vi "PC main.vi"() -> ()   [LabVIEW 2021]
uses:
  <vilib>/Platform/TimedLoop/XDataNode/wakeup.ctl
  <vilib>/Platform/TimedLoop/XDataNode/XDNodeRunTimeDep.lvlib
  <vilib>/Platform/TimedLoop/XDataNode/nitl_modes.ctl
  <vilib>/Platform/TimedLoop/XDataNode/timing_clust.ctl
  <vilib>/platform/TimedLoop/XDataNode/XDataNode.xnode
  <vilib>/RTI DDS Toolkit/Library/LVDDS_library.lvlib
  <vilib>/RTI DDS Toolkit/VIs/AdvancedCreateReader_NumI32.vi
  <vilib>/RTI DDS Toolkit/VIs/AdvancedCreateWriter_NumI32.vi
  <vilib>/RTI DDS Toolkit/Types/RTI DDS Advanced Writer Configuration.ctl
  <vilib>/RTI DDS Toolkit/Types/RTI DDS Advanced Reader Configuration.ctl
  <vilib>/RTI DDS Toolkit/VIs/Read_NumI32.vi
  <vilib>/RTI DDS Toolkit/VIs/Write_NumI32.vi
panel:
  in  "Record?":bool
  out "cluster":T1(graph)={"Numeric 4"=27.89473684210526, "Numeric 4"=27.105263157894736, "Numeric 4"=33.68421052631579}
  in  "Lock":bool
  in  "Python On":bool=TRUE
  in  "DDS On":bool
  out "Period":i64
  out "RBF Weights":dbl[](array[numeric])
  out "Robot Env":cluster{dbl[], dbl[]}[](graph)=[{[-0.02870597177988223], [-0.4509645928750905]}, {[-2.0, 2.0, 0.0], [-2.0, -2.0, 2.0]}, {[0.0], [0.0]}, {[0.0, 0.0, 0.0, 0.0, 0.0, 0.0, 0.0, 0.0, 0.0, -0.0, -0.0, -0.0, -0.0, -0.0, -0.0, -0.0, -0.0, -0.0, -0.0, -0.0, -0.0, -0.0, -0.0, -0.0, -0.0, 0.0, 0.0, 0.0, 0.0, 0.0, 0.0, 0.0], [0.0, 0.0, 0.0, 0.0, 0.0, 0.0, 0.0, 0.0, 0.0, 0.0, 0.0, 0.0, 0.0, 0.0, 0.0, 0.0, 0.0, -0.0, -0.0, -0.0, -0.0, -0.0, -0.0, -0.0, -0.0, -0.0, -0.0, -0.0, -0.0, -0.0, -0.0, -0.0]}]
  in  "Manual Control":dbl[](array[slide])=[27.89473684210526, 27.105263157894736, 33.68421052631579] scale=0.0..50.0
  in  "Manual Control":bool=TRUE
  in  "Host Stop":bool
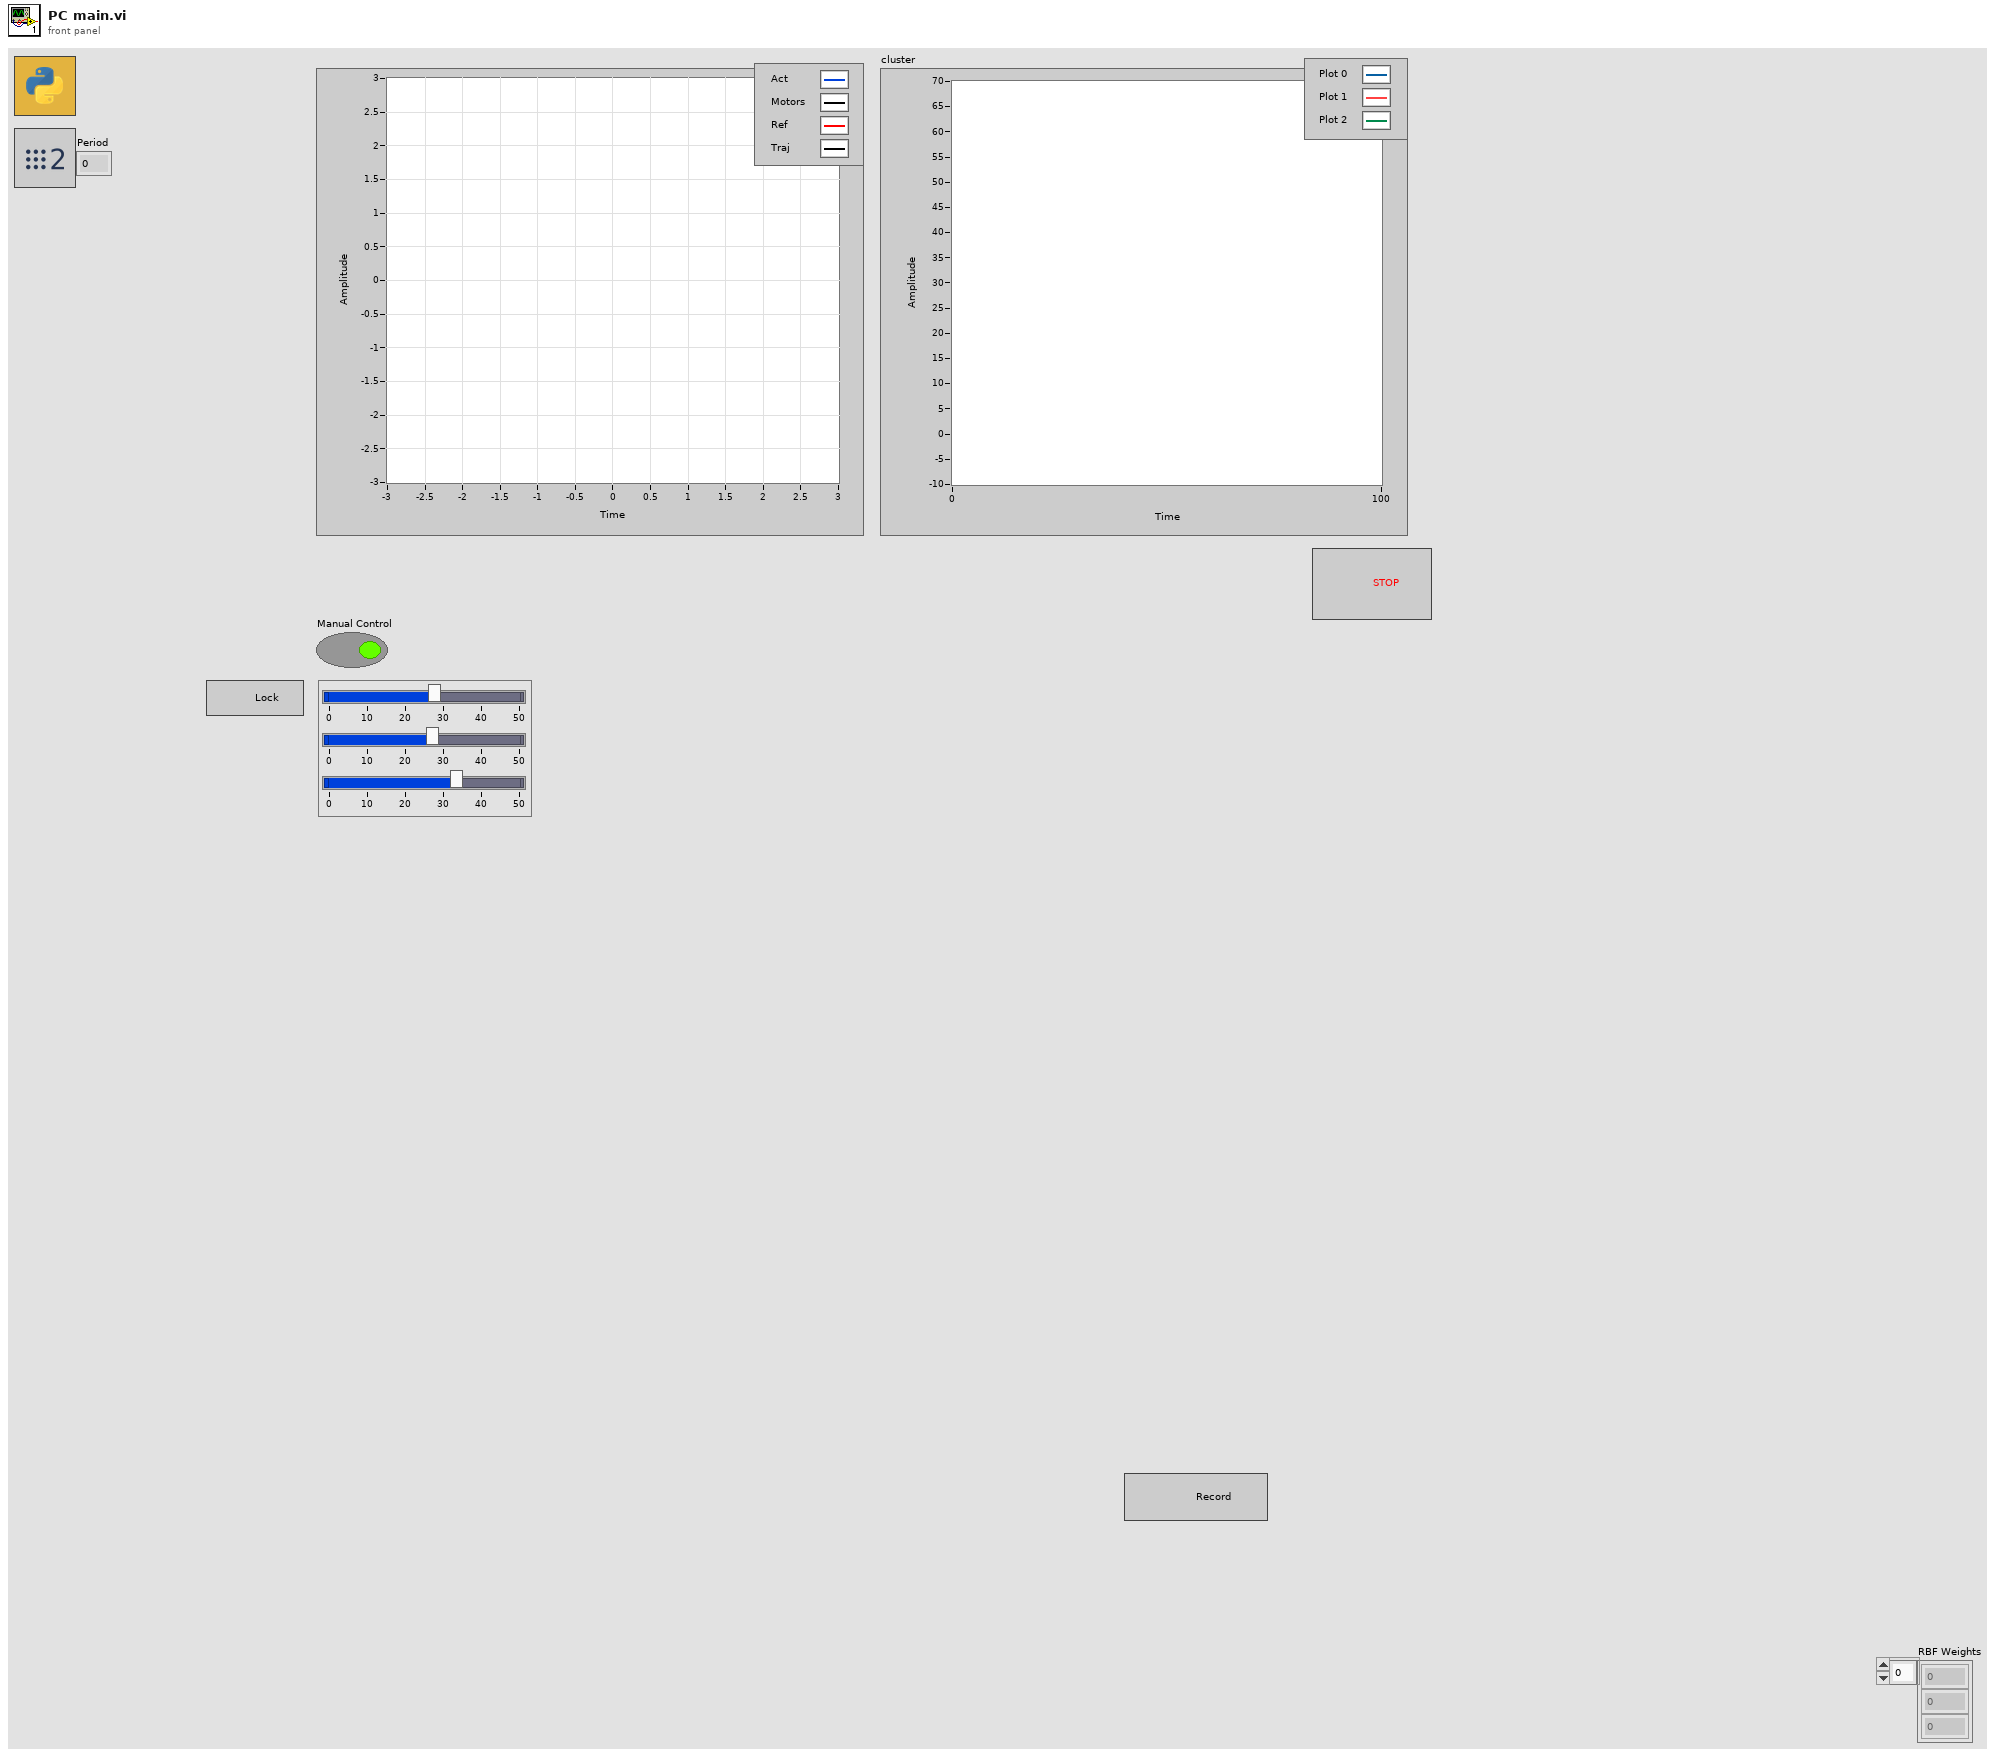
[diagram p1: front panel]
types:
  T1 = cluster{"Numeric 4":dbl, "Numeric 4":dbl, "Numeric 4":dbl}
  T2 = enum16{"open", "open or create", "create or replace", "create", "open (read-only)"}
  T3 = typedef "XDNodeRunTimeDep.lvlib/timing_clust.ctl" = cluster{"Expected End [f-1]":u64, "Actual End [f-1]":u64, "Finished Late? [f-1]":bool, "Expected End [i-1]":u64, "Actual End [i-1]":u64, "Finished Late? [i-1]":bool, "Expected Start [i]":u64, "Actual Start [i]":u64, "Expected Start [f]":u64, "Actual Start [f]":u64, "Source Name":string, "Structure Name":string, "Period":i64, "Deadline":i64, "Offset":i64, "Start":i64, "Priority":i32, "Timeout":i32, "Mode":T4, "Wakeup Reason":T5, "Error":errorcluster, "Source Type":string, "Secondary Source Type":string, "Global End Time":u64, "Global Start Time":u64, "Frame Duration":u64, "Iteration Duration":u64, "Assigned CPU":i32, "I/O Scan Engine Mode":u32}
  T4 = typedef "XDNodeRunTimeDep.lvlib/nitl_modes.ctl" = enum32{"No Change", "Process missed periods, maintain original phase", "Discard missed periods, maintain original phase", "Process missed periods, ignore original phase", "Discard missed periods, ignore original phase"}
  T5 = typedef "XDNodeRunTimeDep.lvlib/wakeup.ctl" = enum32{"Normal", "Aborted", "Asynchronous wakeup", "Timing source error", "Timed loop error", "Timeout"}
  T6 = typedef "LVDDS_library.lvlib/RTI DDS Advanced Reader Configuration.ctl" = cluster{"typeName":string, "keyName":string, "domainParticipantQoSProfile":string, "dataReaderQoSProfile":string, "forceArrayMapping?":bool, "forceExclusiveReader?":bool, "forceRead? (only ExclusiveReader)":bool, "forceUnboundedString?":bool}
  T7 = typedef "LVDDS_library.lvlib/RTI DDS Advanced Writer Configuration.ctl" = cluster{"typeName":string, "keyName":string, "domainParticipantQoSProfile":string, "dataWriterQoSProfile":string, "forceArrayMapping?":bool, "forceUnboundedString?":bool}
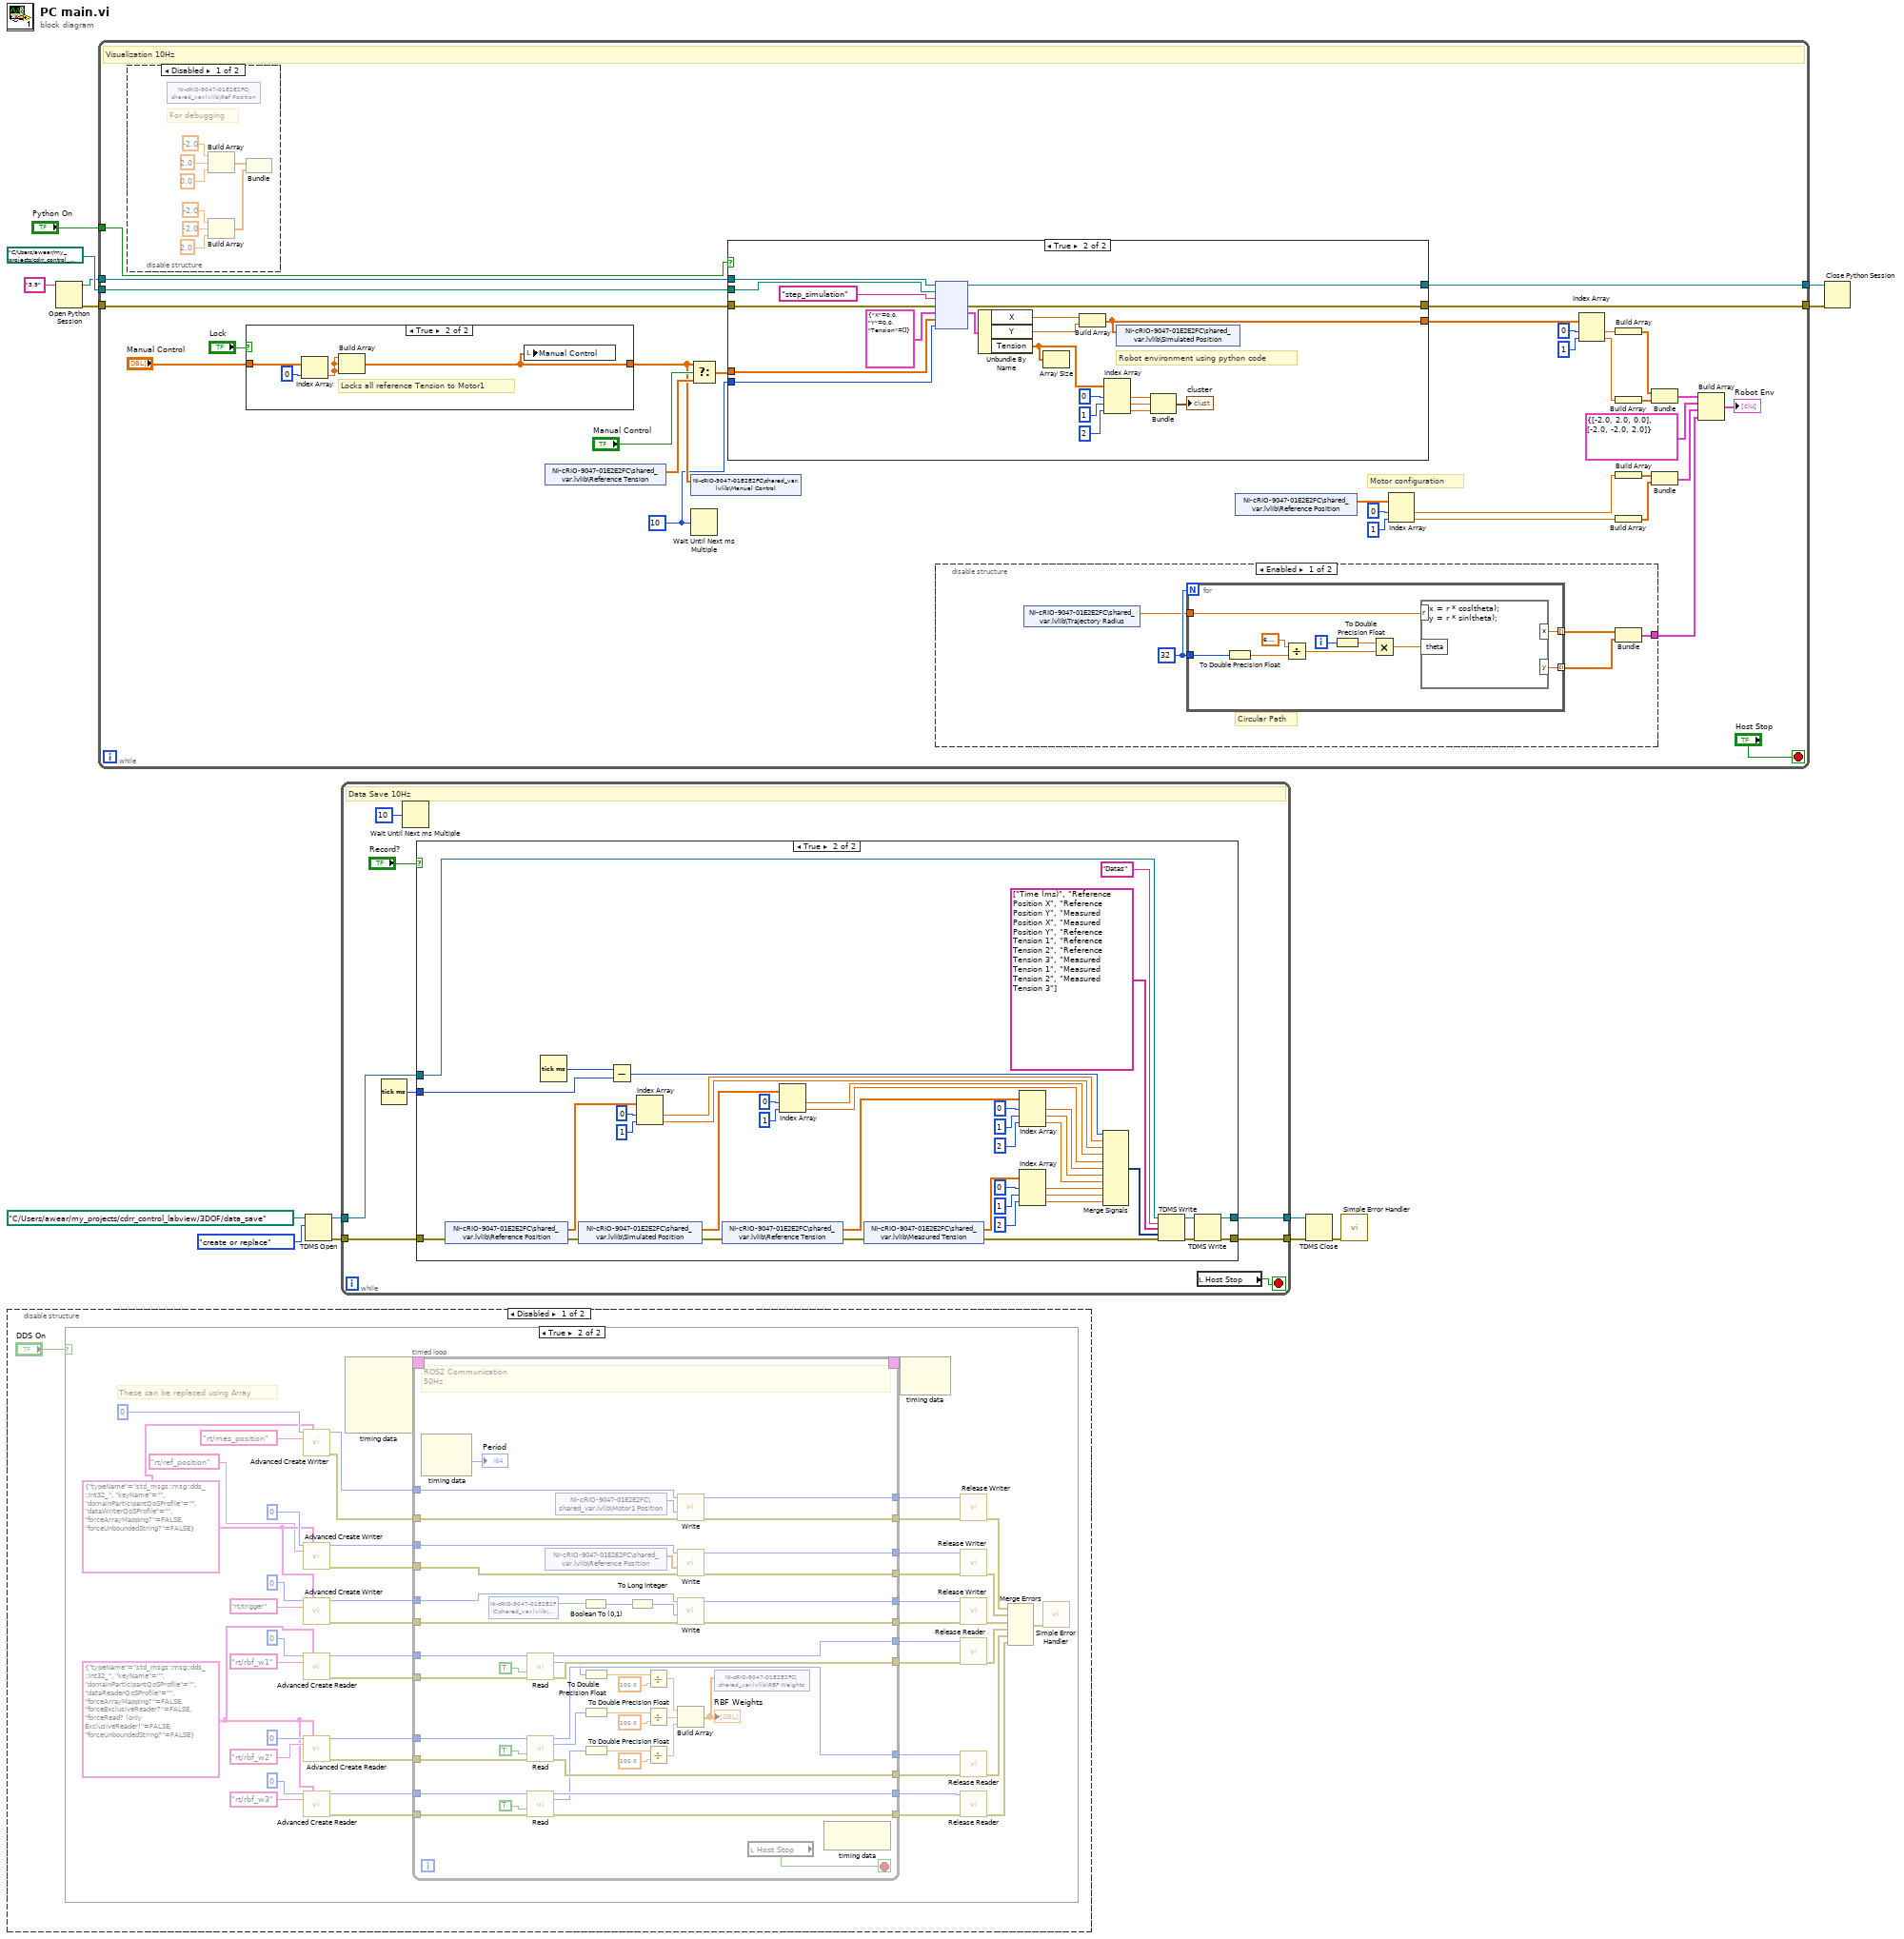
[diagram p0: block diagram]
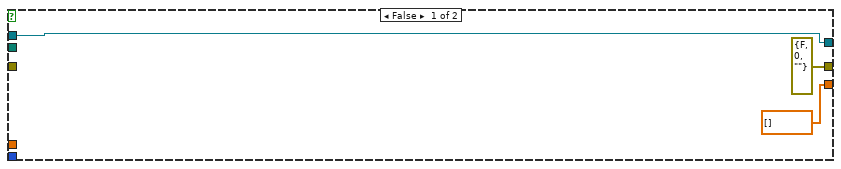
[diagram p5: hidden frame]
diagram:
  n1 = disable-structure shown="Disabled" {
    frame Disabled {
      n2 = case shown="True" "DDS On" {
        frame False {
        }
        frame True {
          w37 = T6 {"typeName"="std_msgs::msg::dds_::Int32_", "keyName"="", "domainParticipantQoSProfile"="", "dataReaderQoSProfile"="", "forceArrayMapping?"=FALSE, "forceExclusiveReader?"=FALSE, "forceRead? (only ExclusiveReader)"=FALSE, "forceUnboundedString?"=FALSE} ("Advanced Reader Configuration 3")
          w25 = T7 {"typeName"="std_msgs::msg::dds_::Int32_", "keyName"="", "domainParticipantQoSProfile"="", "dataWriterQoSProfile"="", "forceArrayMapping?"=FALSE, "forceUnboundedString?"=FALSE} ("Advanced Writer Configuration")
          # "These can be replaced using Array"
          n3 = call-poly <vilib>:"Advanced Create Writer.vi"("Domain Id"=u32 0, "Advanced Writer Configuration"=w25, "Topic Name"="rt/mes_position") -> ("DDS Object Ref"=w29:u64, "error out"=w30:errorcluster)  [unwired: 11 in]
          n4 = call-poly <vilib>:"Advanced Create Writer.vi"("Domain Id"=u32 0, "Advanced Writer Configuration"=w25, "Topic Name"="rt/ref_position") -> ("DDS Object Ref"=w32:u64, "error out"=w31:errorcluster)  [unwired: 11 in]
          n5 = call-poly <vilib>:"Advanced Create Writer.vi"("Domain Id"=u32 0, "Advanced Writer Configuration"=w25, "Topic Name"="rt/trigger") -> ("DDS Object Ref"=w58:u64, "error out"=w59:errorcluster)  [unwired: 11 in]
          n6 = call-poly <vilib>:"Advanced Create Reader.vi"("Domain Id"=u32 0, "Advanced Reader Configuration"=w37, "Topic Name"="rt/rbf_w1") -> ("DDS Object Ref"=w40:u64, "error out"=w41:errorcluster)  [unwired: 11 in]
          n7 = call-poly <vilib>:"Advanced Create Reader.vi"("Domain Id"=u32 0, "Advanced Reader Configuration"=w37, "Topic Name"="rt/rbf_w2") -> ("DDS Object Ref"=w47:u64, "error out"=w46:errorcluster)  [unwired: 11 in]
          n8 = call-poly <vilib>:"Advanced Create Reader.vi"("Domain Id"=u32 0, "Advanced Reader Configuration"=w37, "Topic Name"="rt/rbf_w3") -> ("DDS Object Ref"=w52:u64, "error out"=w53:errorcluster)  [unwired: 11 in]
          n9 = node-c288() -> (w62:T3)  [unwired: 4 in]
          n10 = timed-loop {
            tunnel: w58 -> [w108]
            tunnel: [w107] -> w57
            tunnel: w59 -> [w109]
            tunnel: [w106] -> w56
            tunnel: w53 -> [w105]
            tunnel: [w102] -> w50
            tunnel: w52 -> [w104]
            tunnel: [w103] -> w51
            tunnel: w46 -> [w98]
            tunnel: [w101] -> w49
            tunnel: w47 -> [w99]
            tunnel: [w100] -> w48
            tunnel: w41 -> [w97]
            tunnel: [w94] -> w38
            tunnel: w40 -> [w96]
            tunnel: [w95] -> w39
            tunnel: w32 -> [w91]
            tunnel: [w92] -> w33
            tunnel: w31 -> [w90]
            tunnel: [w93] -> w34
            tunnel: w29 -> [w88]
            tunnel: [w87] -> w28
            tunnel: w30 -> [w89]
            tunnel: [w86] -> w27
            timing: w62 -> [_]
            timing-out: [_] -> w61
            stop <- w84 stop-if-true
            # "ROS2 Communication \n50Hz"
            n11 = node-c288() -> (→"Period":i64)  [unwired: 1 in, 1 out]
            n12 = shared-variable "NI-cRIO-9047-01E2E2FC\\shared_var.lvlib\\Trigger"() -> (w82:bool)  [unwired: 1 in, 1 out]
            n13 = call-poly <vilib>:"Read.vi"("DDS Object Ref in"=w96, "Only New Samples"=TRUE, "error in (no error)"=w97) -> ("DDS Object Ref out"=w95:u64, "Data"=w70:i32, "error out"=w94:errorcluster)  [unwired: 8 in, 2 out]
            n14 = call-poly <vilib>:"Read.vi"("DDS Object Ref in"=w99, "Only New Samples"=TRUE, "error in (no error)"=w98) -> ("DDS Object Ref out"=w100:u64, "Data"=w71:i32, "error out"=w101:errorcluster)  [unwired: 8 in, 2 out]
            n15 = call-poly <vilib>:"Read.vi"("DDS Object Ref in"=w104, "Only New Samples"=TRUE, "error in (no error)"=w105) -> ("DDS Object Ref out"=w103:u64, "Data"=w69:i32, "error out"=w102:errorcluster)  [unwired: 8 in, 2 out]
            n16 = shared-variable "NI-cRIO-9047-01E2E2FC\\shared_var.lvlib\\Reference Position"() -> (w64:dbl[])  [unwired: 1 in, 1 out]
            n17 = shared-variable "NI-cRIO-9047-01E2E2FC\\shared_var.lvlib\\Motor1 Position"() -> (w63:i32)  [unwired: 1 in, 1 out]
            n18 = Boolean To (0,1)(Boolean=w82) -> (0, 1=w81:i16)
            n19 = To Double Precision Float(number=w70) -> (double precision float=w73:dbl)
            n20 = To Double Precision Float(number=w71) -> (double precision float=w76:dbl)
            n21 = To Double Precision Float(number=w69) -> (double precision float=w79:dbl)
            n22 = To Long Integer(number=w81) -> (32bit integer=w80:i32)
            n23 = Divide(x=w73, y=100.0) -> (x/y=w68:dbl)
            n24 = Divide(x=w76, y=100.0) -> (x/y=w67:dbl)
            n25 = Divide(x=w79, y=100.0) -> (x/y=w66:dbl)
            n26 = call-poly <vilib>:"Write.vi"("error in (no error)"=w89, "Data"=w63, "DDS Object Ref in"=w88) -> ("error out"=w86:errorcluster, "DDS Object Ref out"=w87:u64)  [unwired: 7 in]
            n27 = call-poly <vilib>:"Write.vi"("error in (no error)"=w90, "Data"=w64, "DDS Object Ref in"=w91) -> ("error out"=w93:errorcluster, "DDS Object Ref out"=w92:u64)  [unwired: 7 in]
            n28 = call-poly <vilib>:"Write.vi"("error in (no error)"=w109, "Data"=w80, "DDS Object Ref in"=w108) -> ("error out"=w106:errorcluster, "DDS Object Ref out"=w107:u64)  [unwired: 7 in]
            n29 = Build Array(w68, w67, w66) -> (w65:dbl[])
            "RBF Weights" <- w65
            n30 = shared-variable "NI-cRIO-9047-01E2E2FC\\shared_var.lvlib\\RBF Weights"(w65) -> ()  [unwired: 1 in, 1 out]
            n31 = local read "Host Stop"() -> (w84:bool)
            n32 = node-c288() -> ()  [unwired: 1 in, 1 out]
          }
          n33 = node-c288(w61) -> ()  [unwired: 1 out]
          n34 = call <vilib>:"Release Writer.vi"("error in (no error)"=w27, "DDS Object Ref"=w28) -> ("error out"=w21:errorcluster)  [unwired: 9 in]
          n35 = call <vilib>:"Release Writer.vi"("error in (no error)"=w34, "DDS Object Ref"=w33) -> ("error out"=w20:errorcluster)  [unwired: 9 in]
          n36 = call <vilib>:"Release Writer.vi"("error in (no error)"=w56, "DDS Object Ref"=w57) -> ("error out"=w19:errorcluster)  [unwired: 9 in]
          n37 = call <vilib>:"Release Reader.vi"("error in (no error)"=w38, "DDS Object Ref"=w39) -> ("error out"=w18:errorcluster)  [unwired: 9 in]
          n38 = call <vilib>:"Release Reader.vi"("error in (no error)"=w49, "DDS Object Ref"=w48) -> ("error out"=w17:errorcluster)  [unwired: 9 in]
          n39 = call <vilib>:"Release Reader.vi"("error in (no error)"=w50, "DDS Object Ref"=w51) -> ("error out"=w16:errorcluster)  [unwired: 9 in]
          n40 = Merge Errors(w21, w20, w19, w18, w17, w16) -> (w22:errorcluster)
          n41 = call <vilib>:"Simple Error Handler.vi"("error in (no error)"=w22) -> ()  [unwired: 4 in, 5 out]
        }
      }
    }
    frame Enabled {
    }
  }
  n42 = Open Python Session(python version="3.9" ("Python version")) -> (session out=w10:refnum<k35>, error out=w9:errorcluster)  [unwired: 2 in]
  n43 = while {
    tunnel: w10 -> [w144]
    tunnel: [w147] -> w13
    tunnel: w9 -> [w146]
    tunnel: [w145] -> w11
    tunnel: path "C:/Users/awear/my_projects/cdrr_control_labview/Host PC/robot_env.py" ("module path") -> [w143]
    tunnel: "Python On" -> [w138]
    stop <- "Host Stop" stop-if-true
    w115 = u32 10 ("Period 2")
    # "Motor configuration"
    # "Visualization 10Hz"
    n44 = disable-structure shown="Disabled" {
      frame Disabled {
        # "For debugging"
        n45 = shared-variable "NI-cRIO-9047-01E2E2FC\\shared_var.lvlib\\Ref Position"() -> ()  [unwired: 1 in, 2 out]
        n46 = Build Array(-2.0 ("Y"), 2.0 ("Y"), 0.0 ("Y")) -> (w198:dbl[])
        n47 = Build Array(-2.0 ("Y"), -2.0 ("Y"), 2.0 ("Y")) -> (w199:dbl[])
        n48 = Bundle(w198, w199) -> ()  [unwired: 1 in, 1 out]
      }
      frame Enabled {
      }
    }
    n49 = case shown="True" "Lock" {
      tunnel: "Manual Control" -> [w163 w166]
      tunnel: [w163 w164] -> w132
      frame False {
      }
      frame True {
        # "Locks all reference Tension to Motor1"
        n50 = Index Array(array=w166, index=0) -> (element=w165:dbl)
        n51 = Build Array(w165, w165, w165) -> (w164:dbl[])
        n52 = local write "Manual Control"(w164) -> ()
      }
    }
    n53 = shared-variable "NI-cRIO-9047-01E2E2FC\\shared_var.lvlib\\Reference Tension"() -> (w136:dbl[])  [unwired: 1 in, 1 out]
    n54 = Select(t=w132, s="Manual Control", f=w136) -> (s? t:f=w135:dbl[])
    n55 = shared-variable "NI-cRIO-9047-01E2E2FC\\shared_var.lvlib\\Manual Control"(w132) -> ()  [unwired: 1 in, 1 out]
    n56 = Wait Until Next ms Multiple(millisecond multiple=w115) -> ()  [unwired: 1 out]
    n57 = case shown="True" w138 {
      tunnel: [w169 w190] -> w147
      tunnel: w146 -> [_ w189]
      tunnel: [errorcluster {"status"=FALSE, "code"=0, "source"=""} ("function name out") w188] -> w145
      tunnel: w144 -> [w169 w187]
      tunnel: w143 -> [_ w186]
      tunnel: w135 -> [_ w184]
      tunnel: w115 -> [_ w183]
      tunnel: [dbl[] [] w171] -> w117
      frame False {
      }
      frame True {
        # "Robot environment using python code"
        n58 = node(w187, w186, "step_simulation" ("function name"), w189, cluster{"X":dbl, "Y":dbl, "Tension":dbl[]} {"X"=0.0, "Y"=0.0, "Tension"=[]} ("return value"), w184, w183) -> (w190:refnum<k35>, w188:errorcluster, w185:cluster{"X":dbl, "Y":dbl, "Tension":dbl[]})  [unwired: 2 in, 2 out]
        n59 = Unbundle By Name(w185) -> ("X"=w173:dbl, "Y"=w172:dbl, "Tension"=w174:dbl[])
        n60 = Array Size(array=w174) -> ()  [unwired: 1 out]
        n61 = Build Array(w173, w172) -> (w171:dbl[])
        n62 = Index Array(array=w174, index #1=0 ("index"), index #2=1 ("index"), index #3=2 ("index")) -> (element #1=w178:dbl, element #2=w177:dbl, element #3=w176:dbl)
        n63 = shared-variable "NI-cRIO-9047-01E2E2FC\\shared_var.lvlib\\Simulated Position"(w171) -> ()  [unwired: 1 in, 1 out]
        n64 = Bundle("Numeric 4"=w178, "Numeric 4"=w177, "Numeric 4"=w176) -> (→"cluster":T1)  [unwired: 1 in]
      }
    }
    n65 = disable-structure shown="Enabled" {
      disable-tunnel: [w149 _] -> w140
      frame Enabled {
        w150 = 32 ("Drawing Samples")
        # "Circular Path"
        n66 = shared-variable "NI-cRIO-9047-01E2E2FC\\shared_var.lvlib\\Trajectory Radius"() -> (w148:dbl)  [unwired: 1 in, 1 out]
        n67 = for {
          N: w150 -> [_]
          tunnel: [w162] -> w152 mode=indexing
          tunnel: [w161] -> w151 mode=indexing
          tunnel: w150 -> [w157]
          tunnel: w148 -> [w153]
          i -> [w158]
          n68 = To Double Precision Float(number=w157) -> (double precision float=w155:dbl)
          n69 = Divide(x=6.283185307179586, y=w155) -> (x/y=w160:dbl)
          n70 = To Double Precision Float(number=w158) -> (double precision float=w156:dbl)
          n71 = Multiply(x=w156, y=w160) -> (x*y=w159:dbl)
          n72 = formula code="x = r * cos(theta);\ny = r * sin(theta);"("r"=w153, "theta"=w159) -> ("x"=w162:dbl, "y"=w161:dbl)
        }
        n73 = Bundle(w152, w151) -> (w149:cluster{dbl[], dbl[]})  [unwired: 1 in]
      }
      frame Disabled {
      }
    }
    n74 = shared-variable "NI-cRIO-9047-01E2E2FC\\shared_var.lvlib\\Reference Position"() -> (w131:dbl[])  [unwired: 1 in, 1 out]
    n75 = Index Array(array=w131, index #1=0 ("index"), index #2=1 ("index")) -> (element #1=w128:dbl, element #2=w127:dbl)
    n76 = Index Array(array=w117, index #1=0 ("index"), index #2=1 ("index")) -> (element #1=w121:dbl, element #2=w120:dbl)
    n77 = Build Array(w121) -> (w119:dbl[])
    n78 = Build Array(w120) -> (w118:dbl[])
    n79 = Build Array(w128) -> (w126:dbl[])
    n80 = Build Array(w127) -> (w125:dbl[])
    n81 = Bundle(w119, w118) -> (w116:cluster{dbl[], dbl[]})  [unwired: 1 in]
    n82 = Bundle(w126, w125) -> (w124:cluster{dbl[], dbl[]})  [unwired: 1 in]
    n83 = Build Array(w116, cluster{dbl[], dbl[]} {[-2.0, 2.0, 0.0], [-2.0, -2.0, 2.0]} ("output cluster"), w124, w140) -> (→"Robot Env":cluster{dbl[], dbl[]}[])
  }
  n84 = TDMS Open(10:T2."create or replace" ("operation (0:open)"), 11:path "C:/Users/awear/my_projects/cdrr_control_labview/3DOF/data_save" ("file path")) -> (0:w3:errorcluster, 3:w7:refnum<k34>)  [unwired: 5 in]
  n85 = while {
    tunnel: w7 -> [w207]
    tunnel: [w204] -> w6
    tunnel: [w205] -> w4
    tunnel: w3 -> [w206]
    stop <- w201 stop-if-true
    # "Data Save 10Hz"
    n86 = Tick Count (ms)() -> (millisecond timer value=w203:u32)
    n87 = Wait Until Next ms Multiple(millisecond multiple=u32 10 ("Period 2")) -> ()  [unwired: 1 out]
    n88 = case shown="True" "Record?" {
      tunnel: w207 -> [w208 w249]
      tunnel: w206 -> [w209 w221]
      tunnel: [w209 w235] -> w205
      tunnel: [w208 w236] -> w204
      tunnel: w203 -> [_ w244]
      frame False {
      }
      frame True {
        n89 = shared-variable "NI-cRIO-9047-01E2E2FC\\shared_var.lvlib\\Reference Position"(error in=w221) -> (w237:dbl[], error out=w220:errorcluster)
        n90 = Tick Count (ms)() -> (millisecond timer value=w246:u32)
        n91 = shared-variable "NI-cRIO-9047-01E2E2FC\\shared_var.lvlib\\Simulated Position"(error in=w220) -> (w228:dbl[], error out=w219:errorcluster)
        n92 = Subtract(x=w246, y=w244) -> (x-y=w243:u32)
        n93 = Index Array(array=w237, index #1=0 ("index"), index #2=1 ("index")) -> (element #1=w232:dbl, element #2=w231:dbl)
        n94 = shared-variable "NI-cRIO-9047-01E2E2FC\\shared_var.lvlib\\Reference Tension"(error in=w219) -> (w225:dbl[], error out=w214:errorcluster)
        n95 = Index Array(array=w228, index #1=0 ("index"), index #2=1 ("index")) -> (element #1=w227:dbl, element #2=w226:dbl)
        n96 = shared-variable "NI-cRIO-9047-01E2E2FC\\shared_var.lvlib\\Measured Tension"(error in=w214) -> (w215:dbl[], error out=w213:errorcluster)
        n97 = Index Array(array=w225, index #1=0 ("index"), index #2=1 ("index"), index #3=2 ("index")) -> (element #1=w224:dbl, element #2=w223:dbl, element #3=w222:dbl)
        n98 = Index Array(array=w215, index #1=0 ("index"), index #2=1 ("index"), index #3=2 ("index")) -> (element #1=w212:dbl, element #2=w211:dbl, element #3=w210:dbl)
        n99 = Merge Signals(w243, w232, w231, w227, w226, w224, w223, w222, w212, w211, w210) -> (w247:dynamicdata)
        n100 = TDMS Write(0:w249, 5:"Datas" ("group name in (Untitled)"), 7:string[] ["Time (ms)", "Reference Position X", "Reference Position Y", "Measured Position X", "Measured Position Y", "Reference Tension 1", "Reference Tension 2", "Reference Tension 3", "Measured Tension 1", "Measured Tension 2", "Measured Tension 3"] ("channel name(s) in (Untitled)"), 9:w247, 11:w213) -> (4:w234:refnum<k34>, 15:w233:errorcluster)  [unwired: 1 in, 2 out]
        n101 = TDMS Write(0:w234, 11:w233) -> (4:w236:refnum<k34>, 15:w235:errorcluster)  [unwired: 4 in, 2 out]
      }
    }
    n102 = local read "Host Stop"() -> (w201:bool)
  }
  n103 = TDMS Close(8:w4, 11:w6) -> (0:w5:errorcluster)  [unwired: 1 out]
  n104 = call <vilib>:"Simple Error Handler.vi"("error in (no error)"=w5) -> ()  [unwired: 4 in, 5 out]
  n105 = Close Python Session(session in=w13, error in=w11) -> ()  [unwired: 1 out]
